vi "IsHotGoal.vi"(8 "error in":errorcluster, 9 "% Cutoff":dbl, 10 "Num samples":i32) -> (0 "error out":errorcluster, 2 "Hot/Not":bool)   [LabVIEW 2013]
doc: "IsHotGoal checks if the goal is hot at the beginning of autonomous mode.\n-NumSamples determines how many images of the goal the camera will process.\n-% Cutoff (meant to be a decimal value) determines the minimum ratio of hot images/total images needed for IsHotGoal to report a hot goal."
uses:
  TargetType.ctl
panel:
  in  "Color System":u16(ring)=2 items=["RGB", "HSL", "HSV", "HSI"]
  in  "Score cutoff":dbl=50.0
  out "Distance (ft)":dbl
  out "Scores.State":T1
  in  "Color Components":T2={"Hue"={116.0, 148.0}, "Sat"={152.0, 255.0}, "Val"={237.0, 255.0}} {"Val" scale=0.0..255.0; "Sat" scale=0.0..255.0; "Hue" scale=0.0..255.0 scale format="%#_3g"}
  out "Time (ms)":u32
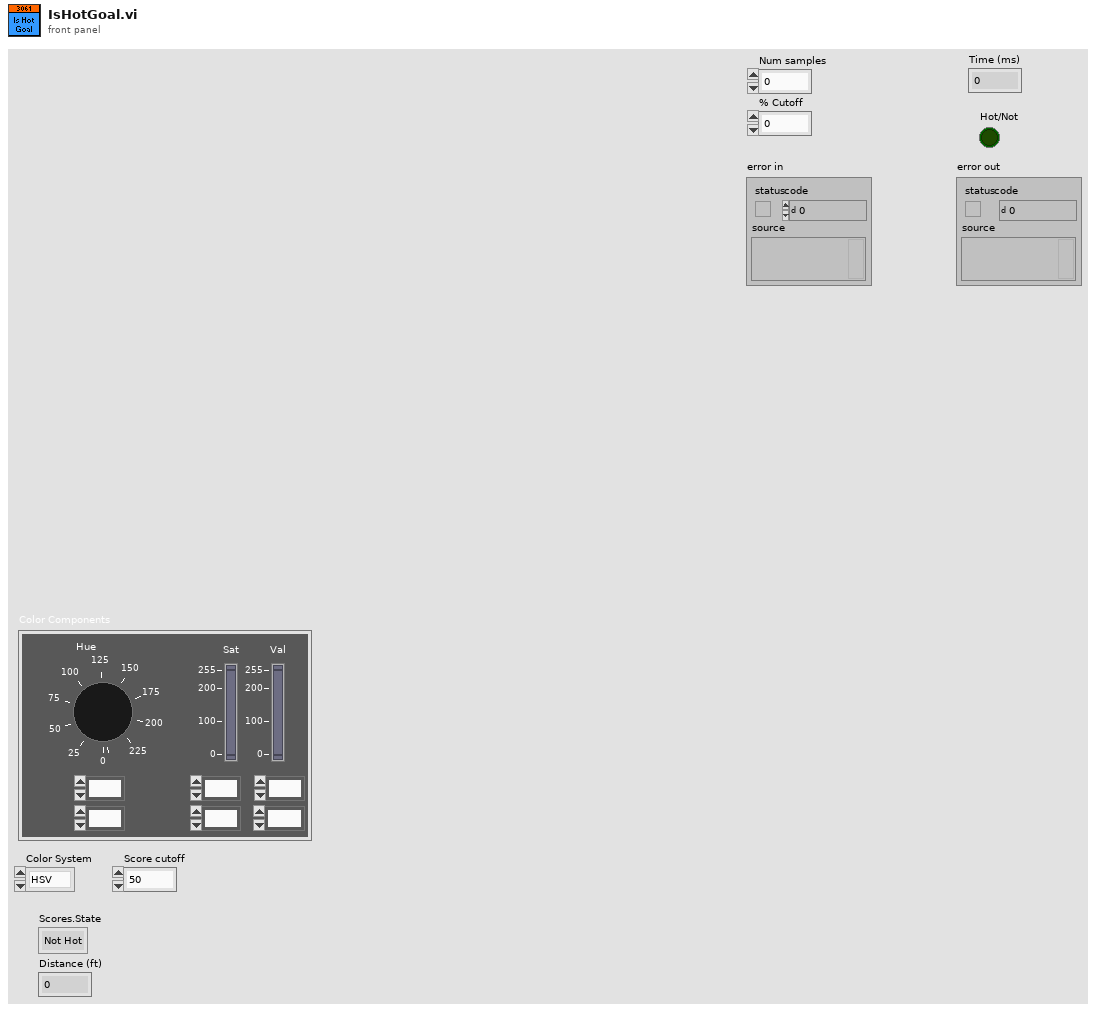
[diagram p1: front panel]
types:
  T1 = typedef "TargetType.ctl" = enum16{"Not Hot", "Hot"}
  T2 = cluster{"Hue":cluster{dbl, dbl}, "Sat":cluster{dbl, dbl}, "Val":cluster{dbl, dbl}}
  T3 = typedef "Image Type" = u32
  T4 = typedef "WPI_CameraDevRef.ctl" = cluster{"Camera Address":string, "CameraStatus":errorcluster, "Acquire Image Notifier":refnum<notifier>}
  T5 = typedef "IMAQ Image.ctl" = refnum<image>
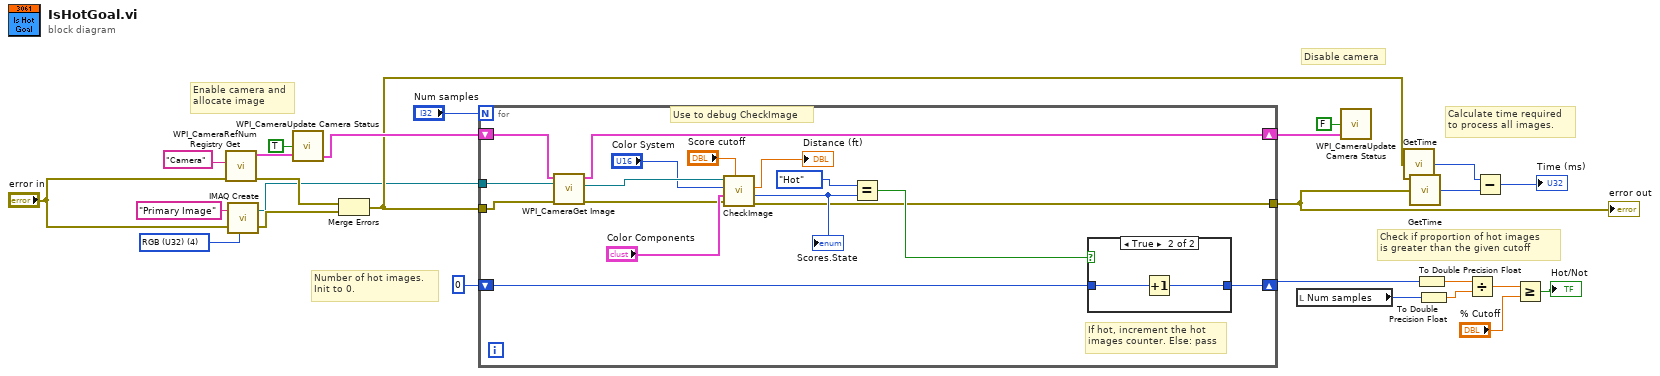
[diagram p0: block diagram]
diagram:
  w9 = T3 4 items=["Grayscale (U8)", "Grayscale (I16)", "Grayscale (SGL)", "Complex (CSG)", "RGB (U32)", "HSL (U32)", "RGB (U64)"] ("Image Type")
  # "Disable camera"
  # "Enable camera and\nallocate image"
  # "Calculate time required \nto process all images."
  # "Check if proportion of hot images\nis greater than the given cutoff"
  # "Number of hot images.\nInit to 0."
  n1 = call <vilib>:"WPI_CameraRefNum Registry Get.vi"("error in (no error)"="error in", "refnum name"="Camera") -> ("error out"=w5:errorcluster, "CameraDevRef"=w12:T4)  [unwired: 8 in]
  n2 = call "IMAQ Create"("Image Name"="Primary Image", "Image Type"=w9, "error in (no error)"="error in") -> ("New Image"=w3:T5, "error out"=w6:errorcluster)  [unwired: 1 in, 1 out]
  n3 = call <vilib>:"WPI_CameraUpdate Camera Status.vi"("CameraDevRef In"=w12, "Enable Vision"=TRUE) -> ("CameraDevRef Out"=w10:T4)  [unwired: 3 in]
  n4 = Merge Errors(w5, w6) -> (w4:errorcluster)
  n5 = for {
    N: "Num samples" -> [_]
    tunnel: w4 -> [w31]
    shift-right: [w41] -> w21
    shift-left: 0 ("Num samples 2") -> [w42]
    tunnel: [w28] -> w15
    tunnel: w3 -> [w32]
    shift-right: [w27] -> w2
    shift-left: w10 -> [w30]
    # "Use to debug CheckImage"
    # "If hot, increment the hot\nimages counter. Else: pass"
    n6 = call <vilib>:"WPI_CameraGet Image.vi"("error in (no error)"=w31, "Image"=w32, "CameraDevRef"=w30) -> ("error out"=w29:errorcluster, "Image Out"=w40:T5, "CameraDevRef Out"=w27:T4)  [unwired: 6 out]
    n7 = call "CheckImage.vi"("Score cutoff"="Score cutoff", "error in"=w29, "Color Components"="Color Components", "Color System"="Color System", "Image"=w40) -> ("error out"=w28:errorcluster, "Scores.State"=w34:T1, "Distance (ft)"=→"Distance (ft)":dbl)  [unwired: 3 in, 1 out]
    "Scores.State" <- w34
    n8 = Equal?(x=TargetType."Hot" ("Scores.State 2"), y=w34) -> (x = y?=w33:bool)
    n9 = case shown="True" w33 {
      tunnel: w42 -> [w43 w45]
      tunnel: [w43 w44] -> w41
      frame False {
      }
      frame True {
        n10 = Increment(x=w45) -> (x+1=w44:i32)
      }
    }
  }
  "error out" <- w15
  n11 = local read "Num samples"() -> (w20:i32)
  n12 = call <vilib>:"WPI_CameraUpdate Camera Status.vi"("CameraDevRef In"=w2, "Enable Vision"=FALSE) -> ()  [unwired: 3 in, 1 out]
  n13 = call "GetTime.vi"("error in"=w4) -> ("Time"=w14:u32)
  n14 = call "GetTime.vi"("error in"=w15) -> ("Time"=w16:u32)
  n15 = To Double Precision Float(number=w21) -> (double precision float=w18:dbl)
  n16 = To Double Precision Float(number=w20) -> (double precision float=w19:dbl)
  n17 = Divide(x=w18, y=w19) -> (x/y=w22:dbl)
  n18 = Subtract(x=w14, y=w16) -> (x-y=→"Time (ms)":u32)
  n19 = Greater Or Equal?(x=w22, y="% Cutoff") -> (x >= y?=→"Hot/Not":bool)
